vi "Increment Calibration Row.vi"(5 "row":i32, 6 "Iteration":i32, 7 "column":i32, 8 "error in (no error)":errorcluster, 10 "NI_report in":refnum<class "NI_report.lvclass">, 11 "Ini File Output in":T1) -> (0 "error out":errorcluster, 2 "Last Row":i32, 3 "Ini File Output out":T1)   [LabVIEW 2015]
doc: "VI usada para incrementar a linha onde são lidos os valores que serão utilizados na calibração."
uses:
  controls/Ini File Output.ctl
  <vilib>/Utility/NIReport.llb/NI_report.lvclass
  <vilib>/addons/_office/NI_ReportGenerationToolkit.lvlib
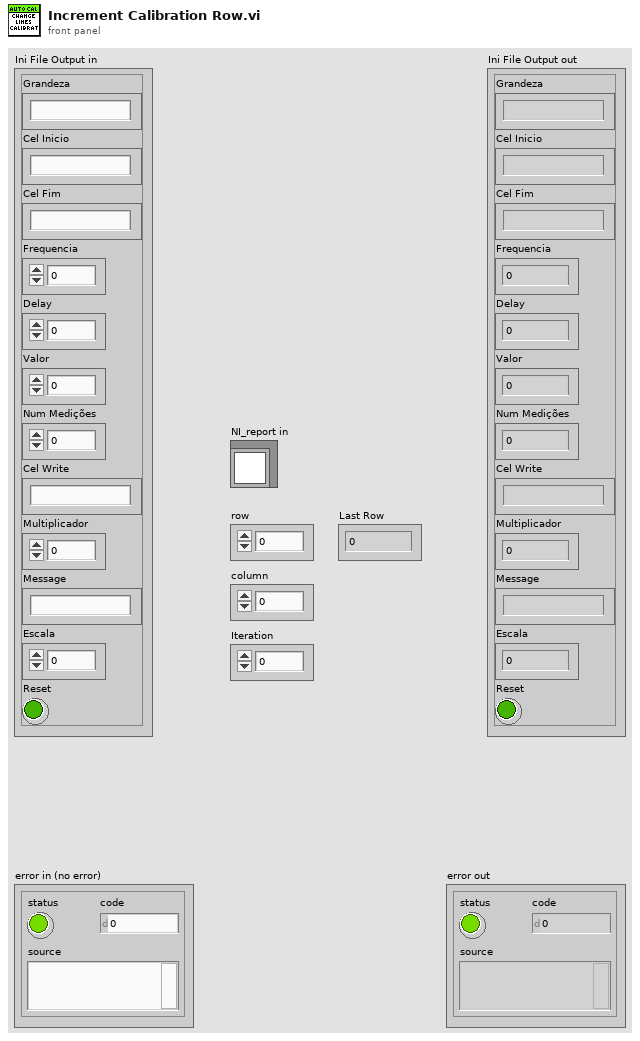
[diagram p1: front panel]
types:
  T1 = typedef "Ini File Output.ctl" = cluster{"Grandeza":string, "Cel Inicio":string, "Cel Fim":string, "Frequencia":dbl, "Delay":dbl, "Valor":dbl, "Num Medições":i32, "Cel Write":string, "Multiplicador":dbl, "Message":string, "Escala":dbl, "Reset":bool}
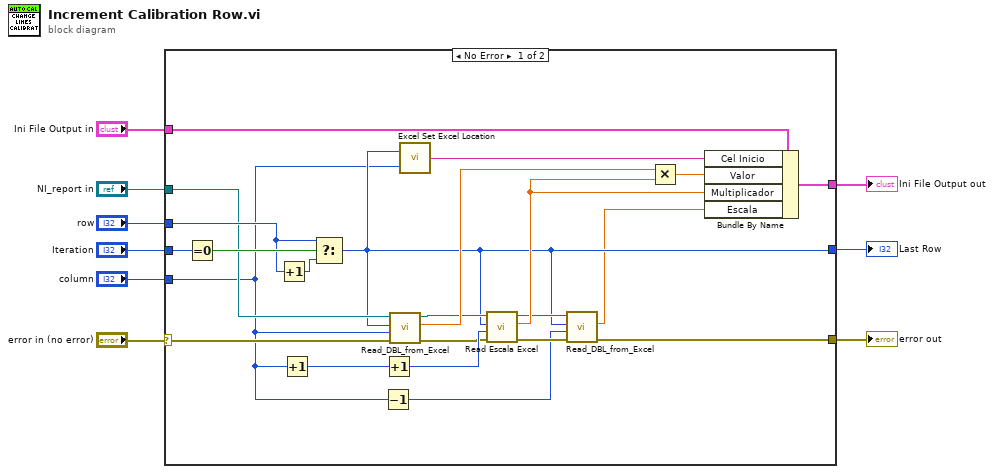
[diagram p0: block diagram]
diagram:
  n1 = case shown="No Error" "error in (no error)" {
    selector: "error in (no error)" -> [w22 w33]
    tunnel: "column" -> [w14 _]
    tunnel: [w15 w34] -> w8
    tunnel: [w11 w33] -> w7
    tunnel: [w31 w35] -> w6
    tunnel: "Ini File Output in" -> [w30 w35]
    tunnel: "Iteration" -> [w29 _]
    tunnel: "row" -> [w26 w34]
    tunnel: "NI_report in" -> [w23 _]
    frame No Error {
      n2 = Equal To 0?(x=w29) -> (x = 0?=w28:bool)
      n3 = Increment(x=w26) -> (x+1=w27:i32)
      n4 = Increment(x=w14) -> (x+1=w10:i32)
      n5 = Select(t=w26, s=w28, f=w27) -> (s? t:f=w15:i32)
      n6 = Decrement(x=w14) -> (x-1=w13:i32)
      n7 = Increment(x=w10) -> (x+1=w25:i32)
      n8 = call "Read_DBL_from_Excel.vi"("error in (no error)"=w22, "Colunm"=w14, "row"=w15, "NI_report in"=w23) -> ("error out"=w21:errorcluster, "data"=w19:dbl, "NI_report Out"=w18:refnum<class "NI_report.lvclass">)  [unwired: 5 in]
      n9 = call <vilib>:"Excel Set Excel Location.vi"("column"=w14, "row"=w15) -> ("cell's name"=w32:string)
      n10 = call "Read Escala Excel.vi"("error in (no error)"=w21, "Colunm"=w25, "row"=w15, "NI_report in"=w18) -> ("error out"=w16:errorcluster, "data"=w20:dbl, "NI_report Out"=w17:refnum<class "NI_report.lvclass">)  [unwired: 5 in]
      n11 = call "Read_DBL_from_Excel.vi"("error in (no error)"=w16, "Colunm"=w13, "row"=w15, "NI_report in"=w17) -> ("error out"=w11:errorcluster, "data"=w12:dbl)  [unwired: 5 in, 1 out]
      n12 = Multiply(x=w19, y=w20) -> (x*y=w24:dbl)
      n13 = Bundle By Name(cluster=w30, "Cel Inicio"=w32, "Valor"=w24, "Multiplicador"=w20, "Escala"=w12) -> (w31:T1)
    }
    frame Error {
    }
  }
  "Last Row" <- w8
  "error out" <- w7
  "Ini File Output out" <- w6
